vi "Get Timeout (ms).vi"(8 "error in (no error)":errorcluster caption="entrée d'erreur (pas d'erreur)", 11 "Wait_OpenFixture en entrée":refnum<class "Remove_Weight.lvclass">) -> (0 "error out":errorcluster caption="sortie d'erreur", 2 "Timeout (ms)":u64, 3 "Wait_OpenFixture en sortie":refnum<class "Remove_Weight.lvclass">)   [LabVIEW 2020, in "Library Test.lvlib" / "Remove_Weight.lvclass"]
uses:
  Remove_Weight.lvclass
  Remove_Weight.lvclass/Remove_Weight.ctl
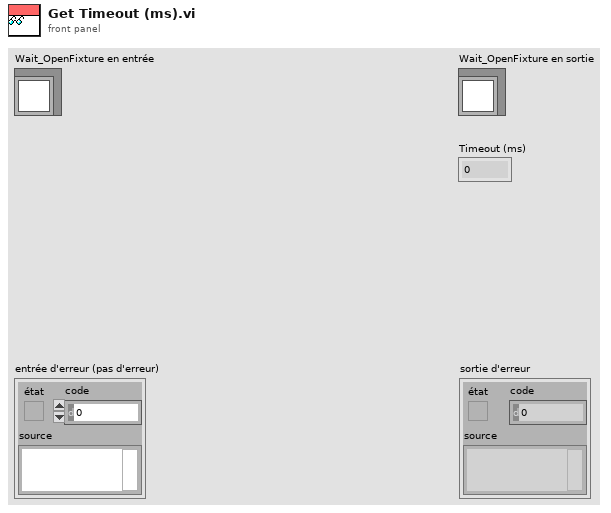
[diagram p1: front panel]
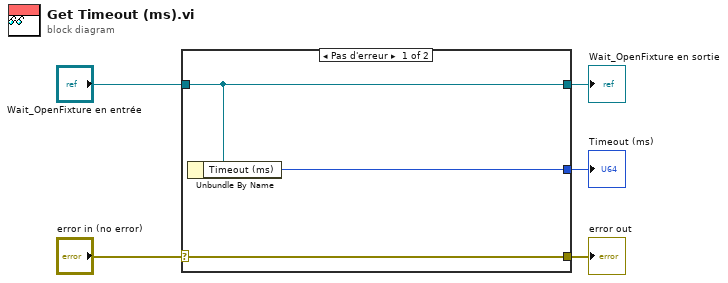
[diagram p0: block diagram]
diagram:
  n1 = case shown="Pas d'erreur" "error in (no error)" {
    selector: "error in (no error)" -> [w8 w9]
    tunnel: [w8 w9] -> w4
    tunnel: [w7 w10] -> w2
    tunnel: "Wait_OpenFixture en entrée" -> [w7 w10]
    tunnel: [w6 _] -> w1
    frame No Error {
      n2 = Unbundle By Name(w7) -> ("Timeout (ms)"=w6:u64)
    }
    frame Error {
    }
  }
  "error out" <- w4
  "Wait_OpenFixture en sortie" <- w2
  "Timeout (ms)" <- w1
